vi "run scripting utility.vi"(8 "error in (no error)":errorcluster, 10 "configuration class path":path, 11 "runtime class path":path) -> (0 "error out":errorcluster)   [LabVIEW 2013]
uses:
  <vilib>/NI/DCAF/Tag Editor Core/control module/script/FromClusterToTagBusScript.vi
  <vilib>/NI/DCAF/Tag Editor Core/control module/script/control module data interface generator.lvlib
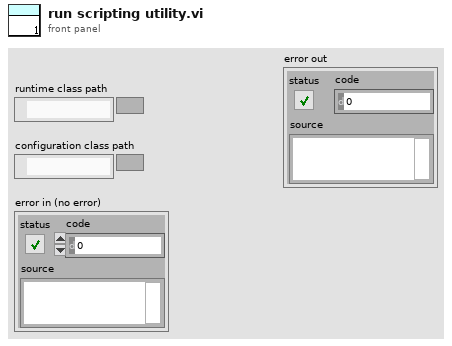
[diagram p1: front panel]
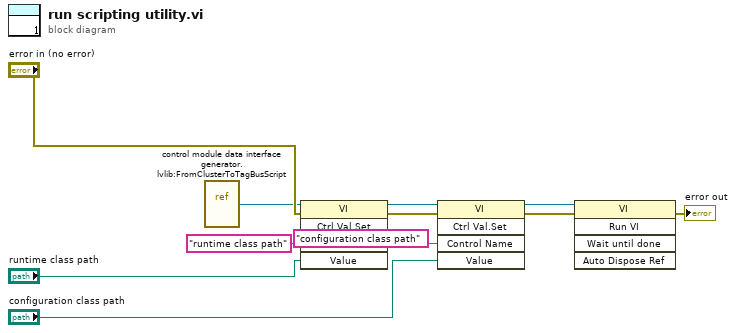
[diagram p0: block diagram]
diagram:
  n1 = vi-ref "control module data interface generator.lvlib:FromClusterToTagBusScript.vi"() -> (w2:refnum<vi>)
  n2 = invoke class="VI" method="Ctrl Val.Set"(reference=w2, error in="error in (no error)", "Control Name"="runtime class path", "Value"="runtime class path") -> (reference out=w8:refnum<vi>, error out=w7:errorcluster)  [unwired: 1 in, 3 out]
  n3 = invoke class="VI" method="Ctrl Val.Set"(reference=w8, error in=w7, "Control Name"="configuration class path", "Value"="configuration class path") -> (reference out=w9:refnum<vi>, error out=w10:errorcluster)  [unwired: 1 in, 3 out]
  n4 = invoke class="VI" method="Run VI"(reference=w9, error in=w10) -> (error out=→"error out":errorcluster)  [unwired: 3 in, 4 out]
